vi "GlobalVariableZadanie11.vi"(6 "Action":enum16{"Set", "Get"}(ring), 11 "input":T1={"Play"=FALSE, "number of samples/ch"=100000, "sound format"={"sample rate (S/s)"=22050.0, "number of channels"=2, "bits per sample"=16}}) -> (3 "output":T1={"Play"=FALSE, "number of samples/ch"=100000, "sound format"={"sample rate (S/s)"=22050.0, "number of channels"=2, "bits per sample"=16}})   [LabVIEW 2020]
uses:
  datacons.ctl
  <vilib>/sound2/lvsound2.llb/Sound Data Format.ctl
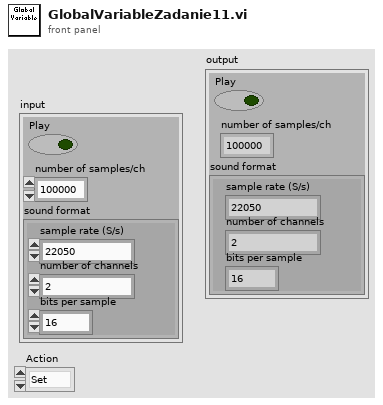
[diagram p1: front panel]
types:
  T1 = typedef "datacons.ctl" = cluster{"Play":bool, "number of samples/ch":i32, "sound format":T2}
  T2 = typedef "Sound Data Format.ctl" = cluster{"sample rate (S/s)":dbl, "number of channels":i32, "bits per sample":i32}
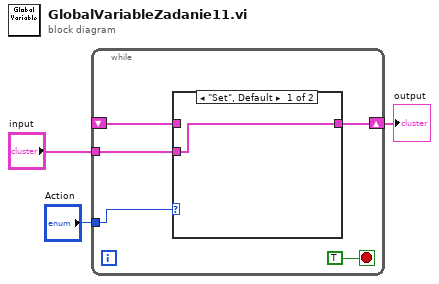
[diagram p0: block diagram]
diagram:
  n1 = while {
    tunnel: "input" -> [w7]
    tunnel: "Action" -> [w8]
    shift-right: [w6] -> w1
    shift-left: _ -> [w5]
    stop <- TRUE stop-if-true
    n2 = case shown="\"Set\", Default" w8 {
      tunnel: w7 -> [w9 _]
      tunnel: [w9 w10] -> w6
      tunnel: w5 -> [_ w10]
      frame "Set", Default {
      }
      frame "Get" {
      }
    }
  }
  "output" <- w1
